vi "testTwoClientsSendEventsAtSameTime.vi"(8 "error in":errorcluster) -> (0 "error out":errorcluster)   [LabVIEW 2018]
uses:
  <vilib>/addons/_JKI Toolkits/Caraya/classes/Assert/Assert Equal Value_Variant.vi
  src/TcpServer/TcpServer.lvclass
  <vilib>/addons/_JKI Toolkits/Caraya/classes/Test/Test.lvclass
  <vilib>/addons/_JKI Toolkits/Caraya/classes/Assert/Assert.lvclass
panel:
  out "Run Server B error":errorcluster
  out "Run Server A error":errorcluster
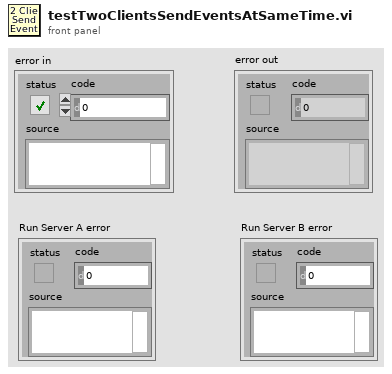
[diagram p1: front panel]
types:
  T1 = cluster{"CmdRead":refnum<user-event>, "EvtRead":refnum<user-event>, "GenRead":refnum<user-event>}
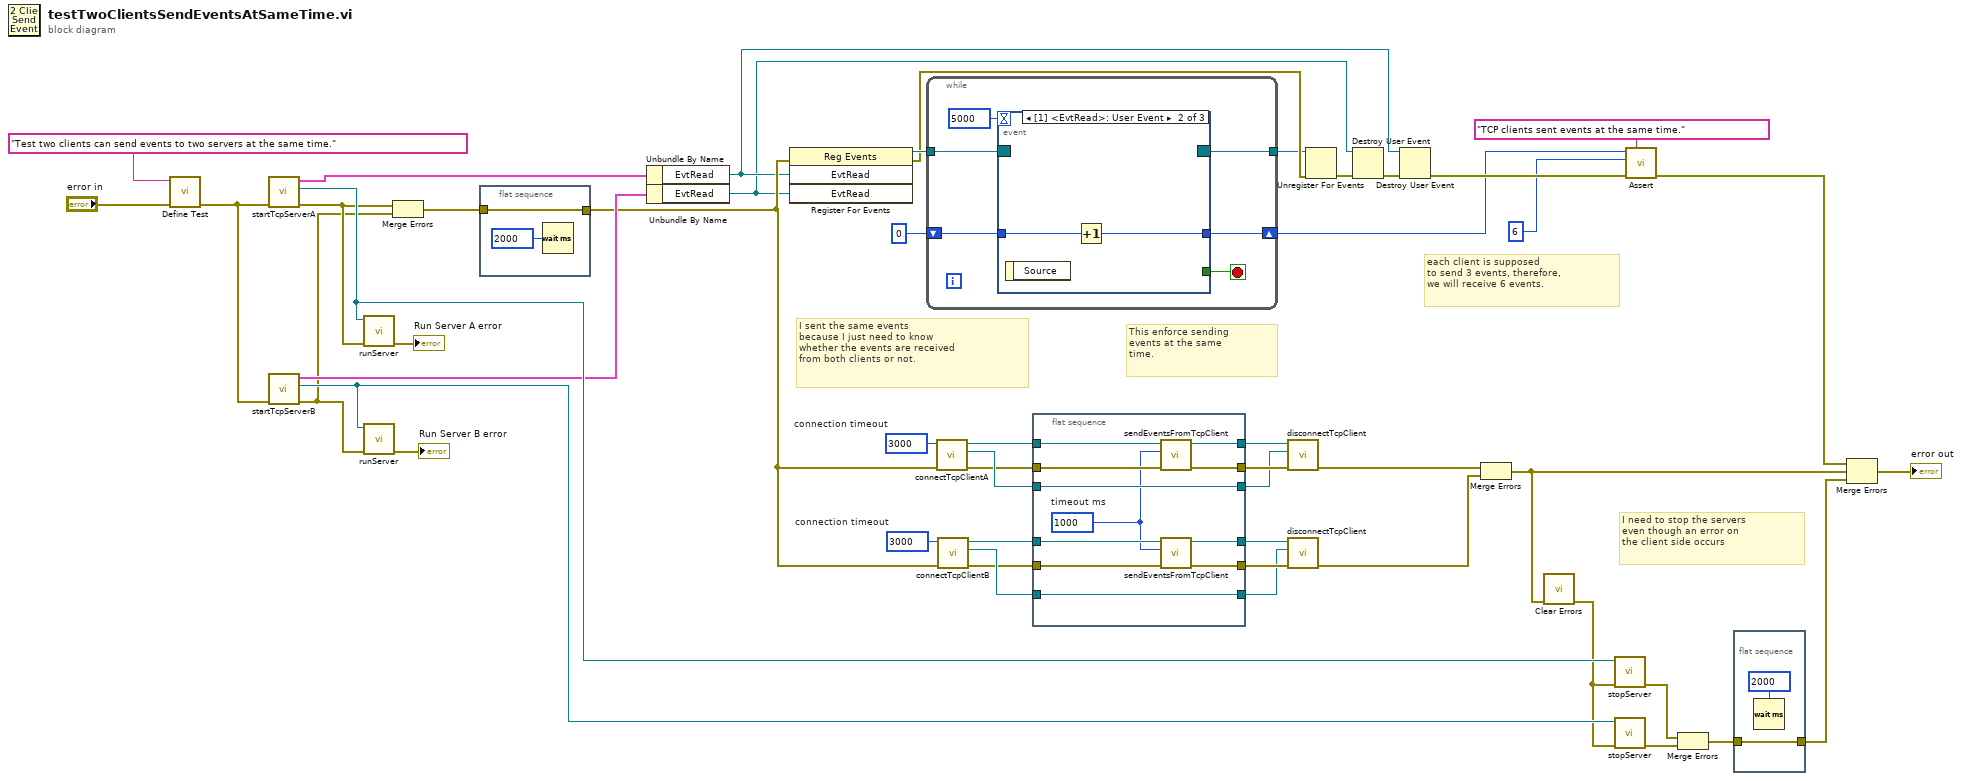
[diagram p0: block diagram]
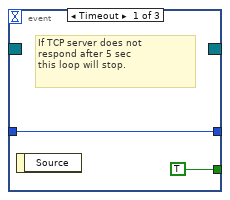
[diagram p2: hidden frame]
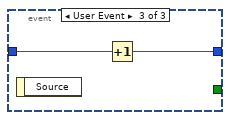
[diagram p3: hidden frame]
diagram:
  w1 = 3000  # connection timeout
  w5 = 3000  # connection timeout
  # "each client is supposed\nto send 3 events, therefore,\nwe will receive 6 events."
  # "I need to stop the servers \neven though an error on \nthe client side occurs"
  # "I sent the same events \nbecause I just need to know\nwhether the events are received \nfrom both clients or not."
  # "This enforce sending\nevents at the same\ntime."
  n1 = call <vilib>:"Define Test.vi"("error in (no error)"="error in", "Label (VI Title)"="Test two clients can send events to two servers at the same time.") -> ("error out"=w32:errorcluster)  [unwired: 9 in]
  n2 = call "startTcpServerA.vi"("error in (no error)"=w32) -> ("error out"=w14:errorcluster, "TcpServer out"=w48:refnum<class "TcpServer.lvclass">, "UserEvents"=w17:T1)  [unwired: 8 in]
  n3 = call "startTcpServerB.vi"("error in (no error)"=w32) -> ("error out"=w12:errorcluster, "TcpServer out"=w25:refnum<class "TcpServer.lvclass">, "UserEvents"=w16:T1)  [unwired: 8 in]
  n4 = call "runServer.vi"("error in (no error)"=w14, "TcpServer in"=w48) -> ("error out (no error)"=→"Run Server A error":errorcluster)  [unwired: 8 in, 1 out]
  n5 = call "runServer.vi"("error in (no error)"=w12, "TcpServer in"=w25) -> ("error out (no error)"=→"Run Server B error":errorcluster)  [unwired: 8 in, 1 out]
  n6 = Merge Errors(w14, w12) -> (w13:errorcluster)
  n7 = flat-sequence {
    tunnel: [w50] -> w15
    tunnel: w13 -> [w50]
    frame #0 {
      n8 = Wait (ms)(milliseconds to wait=u32 2000) -> ()  [unwired: 1 out]
    }
  }
  n9 = Unbundle By Name(w17) -> ("EvtRead"=w7:refnum<user-event>)
  n10 = Unbundle By Name(w16) -> ("EvtRead"=w6:refnum<user-event>)
  n11 = register-events(error in=w15, w7, w6) -> (reference out=w19:refnum<event-registration>, error out=w18:errorcluster)  [unwired: 1 in]
  n12 = while {
    tunnel: w19 -> [w57]
    tunnel: [w56] -> w11
    shift-right: [w52] -> w3
    shift-left: 0 -> [w53]
    stop <- w54 stop-if-true
    n13 = event shown="[1] <EvtRead>: User Event" {
      selector: w57 -> [_ _ _]
      dyn-events: [_ _ _] -> w56
      timeout: 5000 -> [_ _ _]
      tunnel: [TRUE _ _] -> w54
      tunnel: w53 -> [w58 w61 w63]
      tunnel: [w58 w60 w62] -> w52
      event Timeout {
        # "If TCP server does not\nrespond after 5 sec\nthis loop will stop."
        n14 = event-data() -> ()  [unwired: 1 in, 1 out]
      }
      event User Event {
        n15 = event-data() -> ()  [unwired: 1 in, 1 out]
        n16 = Increment(x=w61) -> (x+1=w60:i32)
      }
      event User Event {
        n17 = event-data() -> ()  [unwired: 1 in, 1 out]
        n18 = Increment(x=w63) -> (x+1=w62:i32)
      }
    }
  }
  n19 = call "connectTcpClientA.vi"("error in (no error)"=w15, "connection timeout (ms)"=w5) -> ("error out"=w35:errorcluster, "tel connection ID A out"=w41:refnum<k5>, "cmd connection ID A out"=w42:refnum<k5>)  [unwired: 7 in]
  n20 = call "connectTcpClientB.vi"("error in (no error)"=w15, "timeout ms (5000)"=w1) -> ("error out"=w29:errorcluster, "tel connection ID B out"=w30:refnum<k5>, "cmd connection ID B out"=w31:refnum<k5>)  [unwired: 7 in]
  n21 = flat-sequence {
    tunnel: [w72] -> w39
    tunnel: w42 -> [w73]
    tunnel: [w71] -> w38
    tunnel: [w74] -> w37
    tunnel: w41 -> [w74]
    tunnel: w35 -> [w70]
    tunnel: w31 -> [w68]
    tunnel: [w69] -> w26
    tunnel: w30 -> [w69]
    tunnel: w29 -> [w67]
    tunnel: [w66] -> w28
    tunnel: [w65] -> w27
    frame #0 {
      w64 = 1000  # timeout ms
      n22 = call "sendEventsFromTcpClient.vi"("error in (no error)"=w70, "timeout ms (1000)"=w64, "connectionID"=w73) -> ("error out"=w71:errorcluster, "connectionID"=w72:refnum<k5>)  [unwired: 6 in, 1 out]
      n23 = call "sendEventsFromTcpClient.vi"("error in (no error)"=w67, "timeout ms (1000)"=w64, "connectionID"=w68) -> ("error out"=w65:errorcluster, "connectionID"=w66:refnum<k5>)  [unwired: 6 in, 1 out]
    }
  }
  n24 = call "disconnectTcpClient.vi"("error in (no error)"=w38, "tel connection ID in"=w37, "cmd connection ID in"=w39) -> ("error out"=w36:errorcluster)  [unwired: 8 in]
  n25 = call "disconnectTcpClient.vi"("error in (no error)"=w27, "tel connection ID in"=w26, "cmd connection ID in"=w28) -> ("error out"=w23:errorcluster)  [unwired: 8 in]
  n26 = Unregister For Events(event registration refnum=w11, error in=w18) -> (error out=w10:errorcluster)
  n27 = Destroy User Event(user event=w6, error in=w10) -> (error out=w9:errorcluster)
  n28 = Destroy User Event(user event=w7, error in=w9) -> (error out=w8:errorcluster)
  n29 = Merge Errors(w36, w23) -> (w21:errorcluster)
  n30 = call <vilib>:"Clear Errors.vi"("error in (no error)"=w21) -> ("error out"=w20:errorcluster)  [unwired: 5 in, 1 out]
  n31 = call "stopServer.vi"("error in (no error)"=w20, "tcpServer in"=w48) -> ("error out"=w45:errorcluster)  [unwired: 8 in, 1 out]
  n32 = call "stopServer.vi"("error in (no error)"=w20, "tcpServer in"=w25) -> ("error out"=w44:errorcluster)  [unwired: 8 in, 1 out]
  n33 = call-poly <vilib>:"Assert.vi"("Label"="TCP clients sent events at the same time.", "error in (no error)"=w8, "Y"=6, "X"=w3) -> ("error out"=w24:errorcluster)  [unwired: 7 in]
  n34 = Merge Errors(w45, w44) -> (w43:errorcluster)
  n35 = flat-sequence {
    tunnel: w43 -> [w75]
    tunnel: [w75] -> w22
    frame #0 {
      n36 = Wait (ms)(milliseconds to wait=u32 2000) -> ()  [unwired: 1 out]
    }
  }
  n37 = Merge Errors(w24, w21, w22) -> (→"error out":errorcluster)
